vi "Q8381 Query Wave Data.vi"(2 "set:":u16(ring)=1 items=["Read Y shaft data", "Read X shaft data"], 3 "GPIB address":u16=8 step=1, 4 "VISA resource name":refnum<visa-resource-name>) -> (0 "Received Data":string, 1 "GPIB status":bool)   [LabVIEW 2017]
doc: "Set: 0: Read Y shaft data \n 1: Read X shaft data"
panel:
  out "Data":dbl[](array[numeric]) format="%.5e"
  out "Header":string
  in  "Separater":string=","
  # "Read wave data"
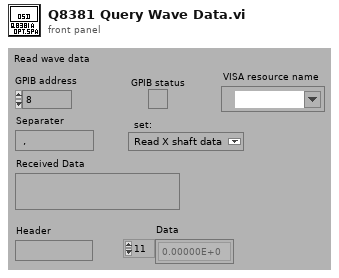
[diagram p1: front panel]
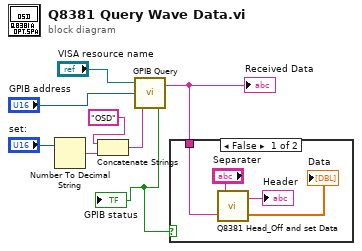
[diagram p0: block diagram]
diagram:
  n1 = Number To Decimal String(number="set:") -> (decimal integer string=w8:string)  [unwired: 1 in]
  n2 = Concatenate Strings("OSD", w8) -> (w2:string)
  n3 = call "GPIB Query.vi"("Command String"=w2, "Address"="GPIB address", "VISA resource name"="VISA resource name") -> ("Error"=w5:bool, "Query Data"=w1:string)
  "GPIB status" <- w5
  "Received Data" <- w1
  n4 = case shown="False" w5 {
    tunnel: w1 -> [w9 _]
    frame False {
      n5 = call "Q8381 Head_Off and set Data.vi"("Input String"=w9, "Separater"="Separater") -> ("Data"=→"Data":dbl[], "Header"=→"Header":string)
    }
    frame True {
    }
  }
